vi "Joysticks.vi"(0 "Enum":enum16{"Start", "Run", "End"}(ring)) -> (1 "Primary Driver":T1, 2 "Secondary Driver":T1)   [LabVIEW 2014]
uses:
  <vilib>/Rock Robotics/WPI/Joystick/WPI_JoystickDeviceEnum.ctl
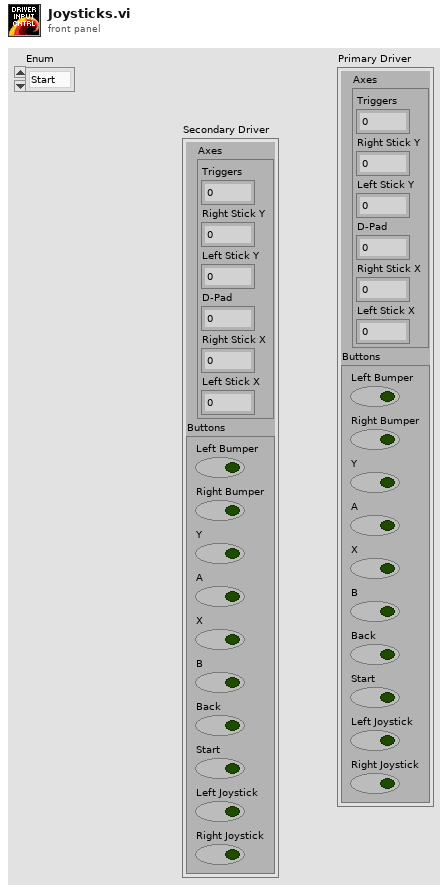
[diagram p1: front panel]
types:
  T1 = cluster{"Axes":cluster{"Triggers":dbl, "Right Stick Y":dbl, "Left Stick Y":dbl, "D-Pad":dbl, "Right Stick X":dbl, "Left Stick X":dbl}, "Buttons":cluster{"Left Bumper":bool, "Right Bumper":bool, "Y":bool, "A":bool, "X":bool, "B":bool, "Back":bool, "Start":bool, "Left Joystick":bool, "Right Joystick":bool}}
  T2 = typedef "WPI_JoystickDeviceEnum.ctl" = enum16{"USB 0", "USB 1", "USB 2", "USB 3", "USB 4", "USB 5"}
  T3 = typedef "WPI_JoystickDevRef.ctl" = cluster{"Device":T2}
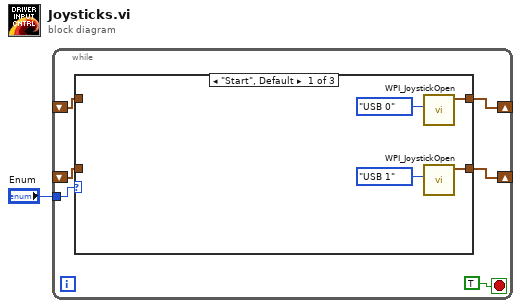
[diagram p0: block diagram]
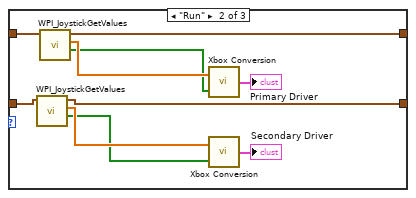
[diagram p2: hidden frame]
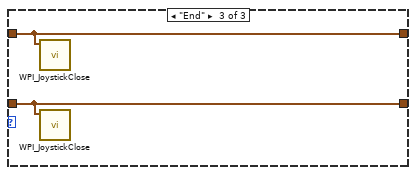
[diagram p3: hidden frame]
diagram:
  n1 = while {
    tunnel: "Enum" -> [w6]
    shift-right: [w4] -> _
    shift-left: _ -> [w5]
    shift-right: [w2] -> _
    shift-left: _ -> [w3]
    stop <- TRUE stop-if-true
    n2 = case shown="\"Start\", Default" w6 {
      tunnel: w5 -> [_ w21 w23]
      tunnel: [w11 w20 w23] -> w4
      tunnel: w3 -> [_ w17 w22]
      tunnel: [w9 w16 w22] -> w2
      frame "Start", Default {
        n3 = call <vilib>:"WPI_JoystickOpen.vi"("JoystickDevice"=WPI_JoystickDeviceEnum."USB 0") -> ("JoystickDevRef"=w11:T3)  [unwired: 10 in]
        n4 = call <vilib>:"WPI_JoystickOpen.vi"("JoystickDevice"=WPI_JoystickDeviceEnum."USB 1") -> ("JoystickDevRef"=w9:T3)  [unwired: 10 in]
      }
      frame "Run" {
        n5 = call <vilib>:"WPI_JoystickGetValues.vi"("JoystickDevRef"=w17) -> ("Buttons"=w12:bool[], "Axes"=w13:dbl[], "JoystickDevRef"=w16:T3)  [unwired: 6 in, 2 out]
        n6 = call <vilib>:"WPI_JoystickGetValues.vi"("JoystickDevRef"=w21) -> ("Buttons"=w14:bool[], "Axes"=w15:dbl[], "JoystickDevRef"=w20:T3)  [unwired: 6 in, 2 out]
        n7 = call "Xbox Conversion.vi"("Buttons"=w14, "Axes"=w15) -> ("Xbox Values"=→"Primary Driver":T1)  [unwired: 1 in]
        n8 = call "Xbox Conversion.vi"("Buttons"=w12, "Axes"=w13) -> ("Xbox Values"=→"Secondary Driver":T1)  [unwired: 1 in]
      }
      frame "End" {
        n9 = call <vilib>:"WPI_JoystickClose.vi"("JoystickDevRef"=w23) -> ()  [unwired: 11 in]
        n10 = call <vilib>:"WPI_JoystickClose.vi"("JoystickDevRef"=w22) -> ()  [unwired: 11 in]
      }
    }
  }
